vi "Device Select.vi"(8 "error in":errorcluster, 10 "SQL query":string="SELECT distinct DeviceName \nFROM\nltt.daq_configuration\n Where ChannelType='Analog_Output' and Enabled=1;", 11 "NI Analog Output in":refnum<class "NI Analog Output.lvclass">) -> (0 "error out":errorcluster, 3 "NI Analog Output out":refnum<class "NI Analog Output.lvclass">)   [LabVIEW 2023, in "HardwareAbstractionLayer_LVOOP.lvlib" / "NI Analog Output.lvclass"]
doc: "This VI Selected Device"
uses:
  NI Analog Output.lvclass
  NI Analog Output.lvclass/NI Analog Output.ctl
  Database/Database.lvclass
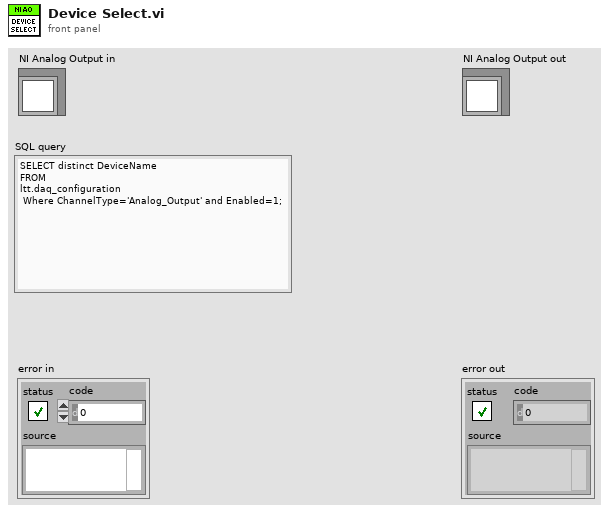
[diagram p1: front panel]
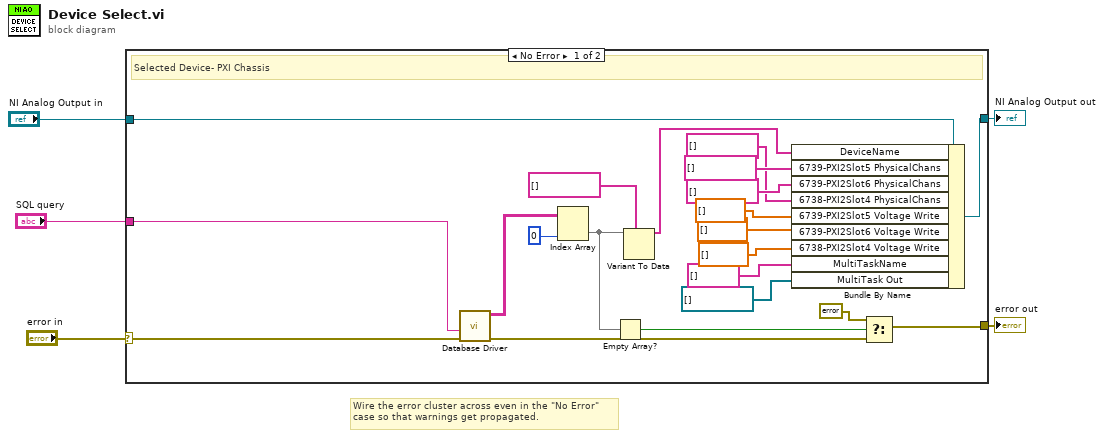
[diagram p0: block diagram]
diagram:
  # "Wire the error cluster across even in the \"No Error\"\ncase so that warnings get propagated."
  n1 = case shown="No Error" "error in" {
    selector: "error in" -> [w20 w28]
    tunnel: [w15 w28] -> w4
    tunnel: [w25 w27] -> w2
    tunnel: "NI Analog Output in" -> [w26 w27]
    tunnel: "SQL query" -> [w19 _]
    frame No Error {
      # "Selected Device- PXI Chassis"
      n2 = call "Database Driver.vi"("error in"=w20, "SQL query"=w19) -> ("error out"=w16:errorcluster, "data"=w21:string[][])  [unwired: 6 in, 2 out]
      n3 = Index Array(array=w21, index (col)=0 ("disabled index (col)")) -> (element=w18:string[])  [unwired: 1 in]
      n4 = Empty Array?(array=w18) -> (empty?=w17:bool)
      n5 = Variant To Data(type=tag[] [] ("DeviceName"), Variant=w18) -> (data=w22:tag[])  [unwired: 1 in, 1 out]
      n6 = Bundle By Name(cluster=w26, "DeviceName"=w22, "6739-PXI2Slot5 PhysicalChans"=tag[] [], "6739-PXI2Slot6 PhysicalChans"=tag[] [], "6738-PXI2Slot4 PhysicalChans"=tag[] [], "6739-PXI2Slot5 Voltage Write"=dbl[] [], "6739-PXI2Slot6 Voltage Write"=dbl[] [], "6738-PXI2Slot4 Voltage Write"=dbl[] [], "MultiTaskName"=string[] [], "MultiTask Out"=refnum<k21>[] []) -> (w25:refnum<class "NI Analog Output.lvclass">)
      n7 = Select(t=errorcluster {"status"=TRUE, "code"=0, "source"="Database does not contains device which is query."}, s=w17, f=w16) -> (s? t:f=w15:errorcluster)
    }
    frame Error {
    }
  }
  "error out" <- w4
  "NI Analog Output out" <- w2
